vi "Write to File.vi"(8 "error in (no error)":errorcluster, 11 "TXT Report":refnum<class "TXT Report.lvclass">) -> (0 "error out":errorcluster, 3 "TXT Report out":refnum<class "TXT Report.lvclass">)   [LabVIEW 2011, in "TXT Report.lvclass"]
doc: "This dynamic dispatch VI takes the information in the object and writes it to a TXT file.\n\nAAL 9/09"
uses:
  TXT Report.lvclass
  Report Class/Report.lvclass
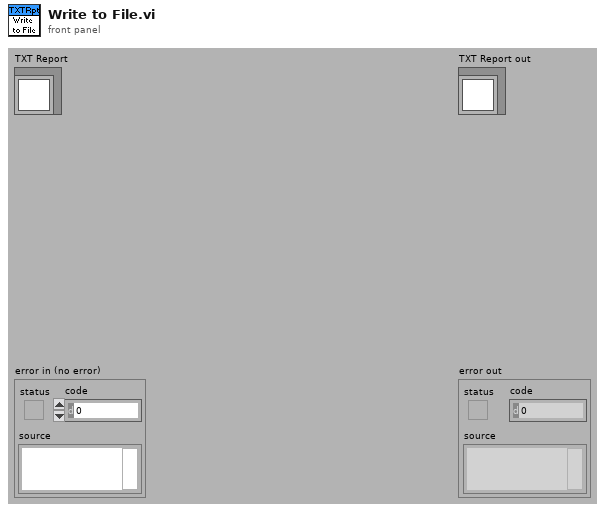
[diagram p1: front panel]
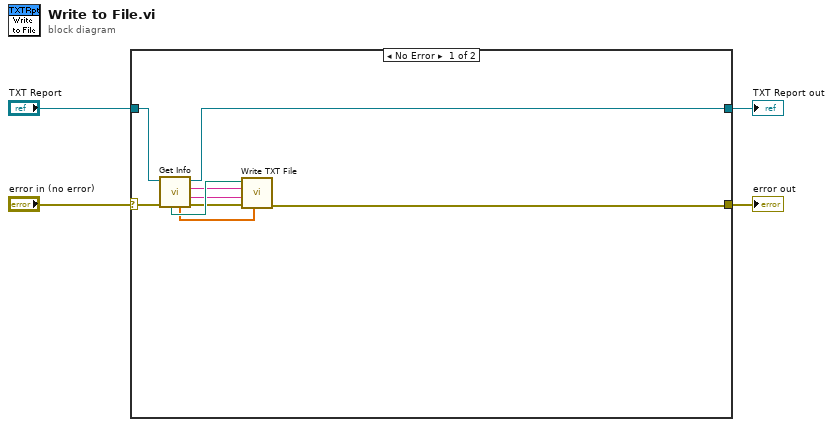
[diagram p0: block diagram]
diagram:
  n1 = case shown="No Error" "error in (no error)" {
    selector: "error in (no error)" -> [w11 w15]
    tunnel: [w5 w15] -> w3
    tunnel: [w12 w14] -> w1
    tunnel: "TXT Report" -> [w13 w14]
    frame No Error {
      n2 = call "Get Info.vi"("error in (no error)"=w11, "Report"=w13) -> ("error out"=w7:errorcluster, "Data & Time String"=w8:string, "Header"=w9:string, "Report out"=w12:refnum<class "TXT Report.lvclass">, "Data Array"=w6:dbl[], "Path"=w10:path)  [unwired: 4 out]
      n3 = call "Write TXT File.vi"("Data Array"=w6, "error in"=w7, "Data & Time String"=w8, "Header"=w9, "Path"=w10) -> ("error out"=w5:errorcluster)  [unwired: 6 in]
    }
    frame Error {
    }
  }
  "error out" <- w3
  "TXT Report out" <- w1
